vi "Get station Seq's paths.vi"(9 "Station":string, 10 "Part Type":string, 11 "Seq Base Path":path) -> (0 "Sys Error Out":errorcluster, 2 "Seq out":string[](array[string]), 3 "Sequence Path":path, 5 "Seqence Info":T1[](array[typedef]))   [LabVIEW 2018]
uses:
  type defs/Sequence Info.ctl
  type defs/Sequence paths.ctl
  type defs/Sequence Status.ctl
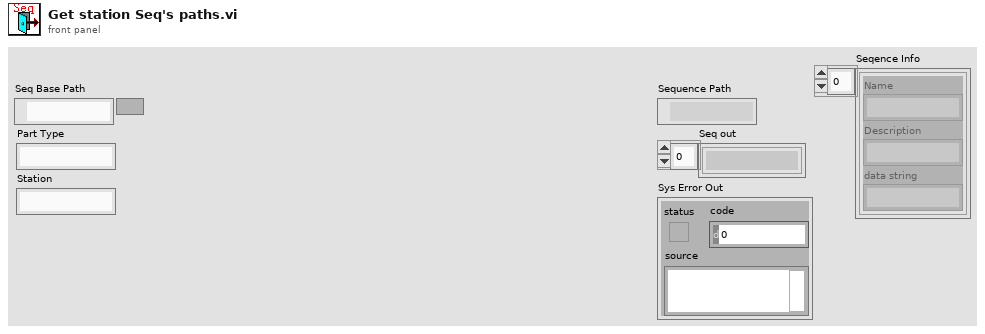
[diagram p1: front panel]
types:
  T1 = typedef "Sequence Info.ctl" = cluster{"Name":string, "Description":string, "data string":string}
  T2 = typedef "Sequence paths.ctl" = cluster{"Sequence Path":path, "Sequence Histroy Path":path, "Current Sequence Path":path, "Sequence Config Path":path, "Sequence VI's Path":path}
  T3 = typedef "Sequence Status.ctl" = enum16{"No Change", "Edited", "New Step", "Deleted", "Moved Up", "Moved Down", "Copied"}
  T4 = cluster{"Paths of Sequence":T2, "Type":string, "Sequence Name:":i32, "Sequence":refnum<vi>, "Steps":refnum<vi>, "Sequence Info":T1[], "Sequence Scroll":u32, "Basic Steps":string[], "Sequences":string[], "Sequence Text":string, "Station":string, "New Step?":bool, "Part Type":string, "User Name":string, "Sequence History":string[][], "Sequence Status":T3, "Sequence History Index":i32, "Step History Data":string[], "VI Names":string[], "Sys Error":errorcluster, "Current Sequence":string[][], "Base Path":path, "Description":string[]}
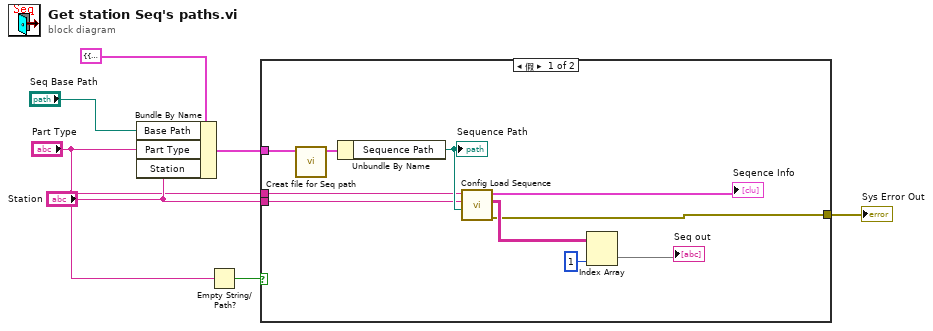
[diagram p0: block diagram]
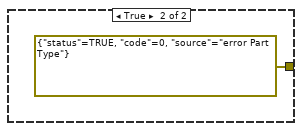
[diagram p2: hidden frame]
diagram:
  n1 = Bundle By Name(cluster=T4 {"Paths of Sequence"={"Sequence Path"=path "", "Sequence Histroy Path"=path "", "Current Sequence Path"=path "", "Sequence Config Path"=path "", "Sequence VI's Path"=path ""}, "Type"="", "Sequence Name:"=0, "Sequence"=refnum, "Steps"=refnum, "Sequence Info"=[], "Sequence Scroll"=0, "Basic Steps"=[], "Sequences"=[], "Sequence Text"="", "Station"="", "New Step?"=FALSE, "Part Type"="", "User Name"="", "Sequence History"=[], "Sequence Status"=enum."No Change", "Sequence History Index"=0, "Step History Data"=[], "VI Names"=[], "Sys Error"={"status"=FALSE, "code"=0, "source"=""}, "Current Sequence"=[], "Base Path"=path "", "Description"=[]} ("ini in"), "Base Path"="Seq Base Path", "Part Type"="Part Type", "Station"="Station") -> (w6:T4)
  n2 = Empty String/Path?(string/path="Part Type") -> (empty?=w1:bool)
  n3 = case shown="假" w1 {
    tunnel: w6 -> [w17 _]
    tunnel: "Part Type" -> [w14 _]
    tunnel: "Station" -> [w13 _]
    tunnel: [w9 errorcluster {"status"=TRUE, "code"=0, "source"="error Part Type"} ("Sys Error Out")] -> w3
    frame False {
      n4 = call "Creat file for Seq path.vi"("ini in"=w17) -> ("Paths of Sequence"=w16:T2)  [unwired: 10 in]
      n5 = Unbundle By Name(w16) -> ("Sequence Path"=w15:path)
      "Sequence Path" <- w15
      n6 = call "Config Load Sequence.vi"("Base Path"=w15, "Station"=w13, "Part Type"=w14) -> ("Sys Error Out"=w9:errorcluster, "Item Names"=w11:string[][], "Seqence Info"=→"Seqence Info":T1[])  [unwired: 5 in, 1 out]
      n7 = Index Array(array=w11, index (col)=1 ("禁用的索引 (列)")) -> (element=→"Seq out":string[])  [unwired: 1 in]
    }
    frame True {
    }
  }
  "Sys Error Out" <- w3
